vi "NPC3SG Convert Calibration v10.6.2.vi"(2 "Calibration File":path, 3 "Is Voltage?":bool, 4 "Axis":u16(ring) items=["X", "Y", "Z"], 5 "Input Value":dbl) -> (0 "Has calibration?":bool, 1 "Output Value":dbl)   [LabVIEW 2010]
uses:
  <vilib>/Utility/file.llb/Read From Spreadsheet File (DBL).vi
panel:
  out "Positions (µm)":dbl[](array[numeric])
  out "Voltages (V)":dbl[](array[numeric])
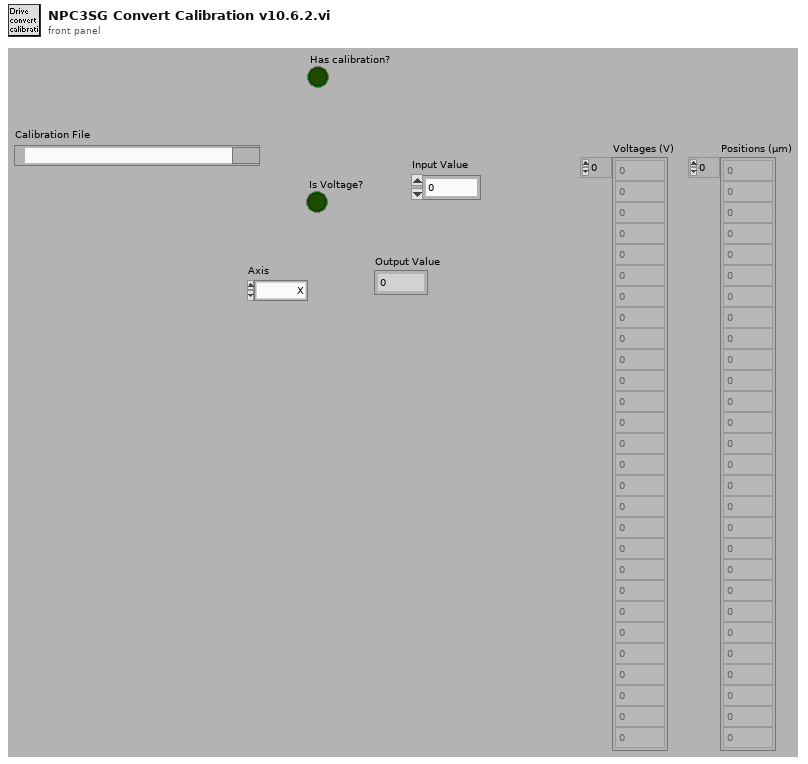
[diagram p1: front panel]
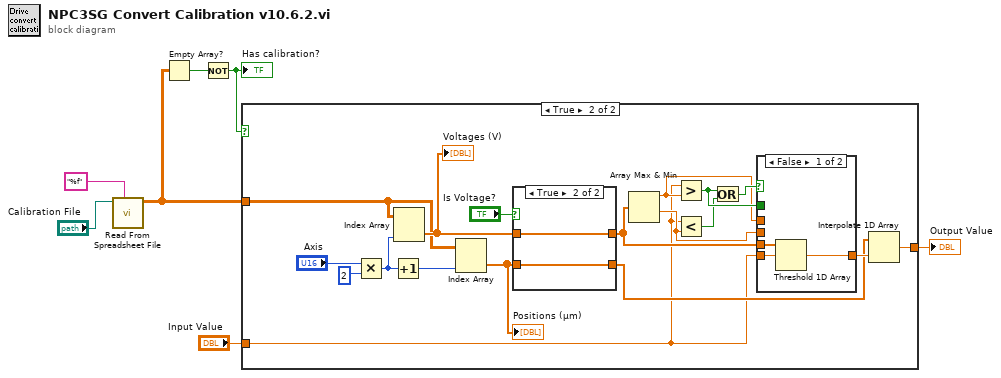
[diagram p0: block diagram]
diagram:
  n1 = call-poly <vilib>:"Read From Spreadsheet File.vi"("format (%.3f)"="%f", "file path (dialog if empty)"="Calibration File") -> ("all rows"=w3:dbl[][])  [unwired: 5 in, 4 out]
  n2 = Empty Array?(array=w3) -> (empty?=w4:bool)
  n3 = Not(x=w4) -> (.not. x?=w2:bool)
  "Has calibration?" <- w2
  n4 = case shown="True" w2 {
    tunnel: [w8 w17] -> w6
    tunnel: "Input Value" -> [w8 w16]
    tunnel: w3 -> [_ w9]
    frame False {
    }
    frame True {
      n5 = Multiply(x="Axis", y=u16 2) -> (x*y=w15:u16)
      n6 = Increment(x=w15) -> (x+1=w14:u16)
      n7 = Index Array(array=w9, index (col)=w15) -> (element=w11:dbl[])  [unwired: 1 in]
      "Voltages (V)" <- w11
      n8 = Index Array(array=w9, index (col)=w14) -> (element=w10:dbl[])  [unwired: 1 in]
      "Positions (µm)" <- w10
      n9 = case shown="True" "Is Voltage?" {
        tunnel: [w36 w39] -> w26
        tunnel: w11 -> [w37 w39]
        tunnel: [w37 w38] -> w21
        tunnel: w10 -> [w36 w38]
        frame False {
        }
        frame True {
        }
      }
      n10 = Array Max & Min(array=w26) -> (max value=w19:dbl, min value=w18:dbl)  [unwired: 2 out]
      n11 = Greater?(x=w16, y=w19) -> (0:w24:bool)
      n12 = Less?(x=w16, y=w18) -> (x < y?=w22:bool)
      n13 = Or(x=w24, y=w22) -> (x .or. y?=w23:bool)
      n14 = case shown="False" w23 {
        tunnel: w24 -> [_ w33]
        tunnel: [w27 w32] -> w25
        tunnel: w26 -> [w29 _]
        tunnel: w16 -> [w28 _]
        tunnel: w19 -> [_ w31]
        tunnel: w18 -> [_ w30]
        frame False {
          n15 = Threshold 1D Array(2:w28, 3:w29) -> (0:w27:dbl)  [unwired: 1 in]
        }
        frame True {
          n16 = case shown="False" w33 {
            tunnel: [w34 w35] -> w32
            tunnel: w31 -> [_ w35]
            tunnel: w30 -> [w34 _]
            frame False {
            }
            frame True {
            }
          }
        }
      }
      n17 = Interpolate 1D Array(1:w25, 2:w21) -> (0:w17:dbl)
    }
  }
  "Output Value" <- w6
